vi "KE6517_Test.vi"(8 "error in (no error)":errorcluster, 11 "KE6517 in":refnum<class "KE6517.lvclass">) -> (0 "error out":errorcluster, 3 "KE6517 out":refnum<class "KE6517.lvclass">)   [LabVIEW 2013, in "KE6517.lvclass"]
uses:
  KE6517.lvclass
  <vilib>/Platform/TimedLoop/XDataNode/timing_clust.ctl
  <vilib>/Platform/TimedLoop/XDataNode/nitl_modes.ctl
  <vilib>/Platform/TimedLoop/XDataNode/wakeup.ctl
  <vilib>/platform/TimedLoop/XDataNode/XDataNode.xnode
  <vilib>/Platform/TimedLoop/XDataNode/XDNodeRunTimeDep.lvlib
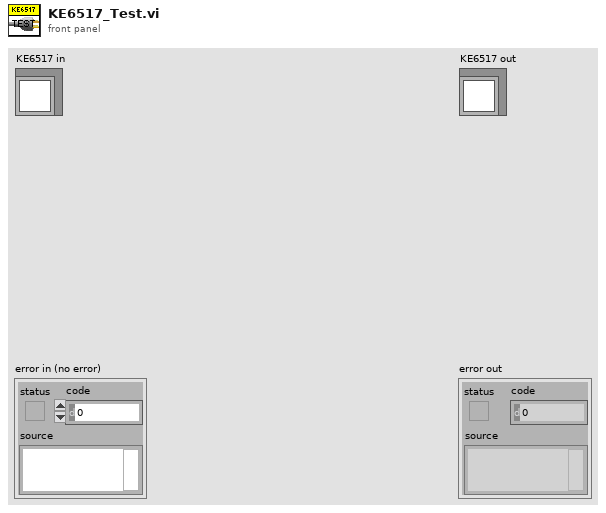
[diagram p1: front panel]
types:
  T1 = typedef "XDNodeRunTimeDep.lvlib/timing_clust.ctl" = cluster{"Expected End [f-1]":u64, "Actual End [f-1]":u64, "Finished Late? [f-1]":bool, "Expected End [i-1]":u64, "Actual End [i-1]":u64, "Finished Late? [i-1]":bool, "Expected Start [i]":u64, "Actual Start [i]":u64, "Expected Start [f]":u64, "Actual Start [f]":u64, "Source Name":string, "Structure Name":string, "Period":i64, "Deadline":i64, "Offset":i64, "Start":i64, "Priority":i32, "Timeout":i32, "Mode":T2, "Wakeup Reason":T3, "Error":errorcluster, "Source Type":string, "Secondary Source Type":string, "Global End Time":u64, "Global Start Time":u64, "Frame Duration":u64, "Iteration Duration":u64, "Assigned CPU":i32, "I/O Scan Engine Mode":u32}
  T2 = typedef "XDNodeRunTimeDep.lvlib/nitl_modes.ctl" = enum32{"No Change", "Process missed periods, maintain original phase", "Discard missed periods, maintain original phase", "Process missed periods, ignore original phase", "Discard missed periods, ignore original phase"}
  T3 = typedef "XDNodeRunTimeDep.lvlib/wakeup.ctl" = enum32{"Normal", "Aborted", "Asynchronous wakeup", "Timing source error", "Timed loop error", "Timeout"}
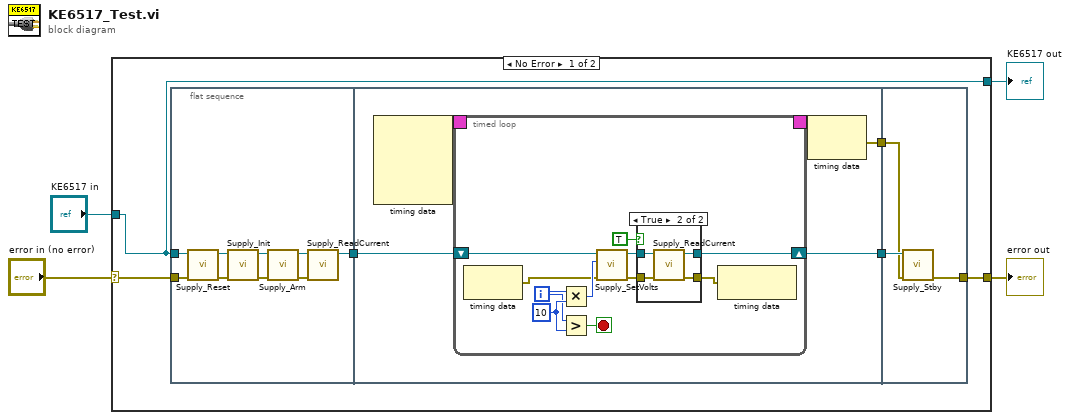
[diagram p0: block diagram]
diagram:
  n1 = case shown="No Error" "error in (no error)" {
    selector: "error in (no error)" -> [w5 w54]
    tunnel: [w7 w54] -> w3
    tunnel: [w6 w53] -> w1
    tunnel: "KE6517 in" -> [w6 w53]
    frame No Error {
      n2 = flat-sequence {
        tunnel: w5 -> [w14]
        tunnel: w6 -> [w13]
        tunnel: [w11] -> w10
        tunnel: w10 -> [w24]
        tunnel: [w23] -> w9
        tunnel: [w20] -> w8
        tunnel: [w50] -> w7
        tunnel: w9 -> [w51]
        tunnel: w8 -> [w52]
        frame #0 {
          n3 = call-dynamic "Supply_Reset.vi"("error in (no error)"=w14, "SupplyControl in"=w13) -> ("error out"=w18:errorcluster, "SupplyControl out"=w12:refnum<class "KE6517.lvclass">)  [unwired: 8 in]
          n4 = call-dynamic "Supply_Init.vi"("error in (no error)"=w18, "SupplyControl in"=w12) -> ("error out"=w17:errorcluster, "SupplyControl out"=w19:refnum<class "KE6517.lvclass">)  [unwired: 8 in]
          n5 = call-dynamic "Supply_Arm.vi"("error in (no error)"=w17, "SupplyControl in"=w19) -> ("error out"=w15:errorcluster, "SupplyControl out"=w16:refnum<class "KE6517.lvclass">)  [unwired: 8 in]
          n6 = call-dynamic "Supply_ReadCurrent.vi"("error in (no error)"=w15, "SupplyControl in"=w16) -> ("SupplyControl out"=w11:refnum<class "KE6517.lvclass">)  [unwired: 7 in, 2 out]
        }
        frame #1 {
          n7 = node-c288() -> (w22:T1)  [unwired: 4 in]
          n8 = timed-loop {
            timing: w22 -> [_]
            timing-out: [_] -> w21
            shift-right: [w32] -> w20
            shift-left: w24 -> [w29]
            i -> [w34]
            stop <- w33 stop-if-true
            w35 = 10
            n9 = node-c288() -> (w27:errorcluster)  [unwired: 1 in]
            n10 = Multiply(x=w34, y=w35) -> (x*y=w28:i32)
            n11 = Greater?(x=w34, y=w35) -> (0:w33:bool)
            n12 = call-dynamic "Supply_SetVolts.vi"("error in (no error)"=w27, "Volts IN [V]"=w28, "KE6517 in"=w29) -> ("error out"=w25:errorcluster, "KE6517 out"=w26:refnum<class "KE6517.lvclass">)  [unwired: 6 in, 1 out]
            n13 = case shown="True" TRUE {
              tunnel: w25 -> [w37 w41]
              tunnel: w26 -> [w36 w40]
              tunnel: [w36 w39] -> w32
              tunnel: [w37 w38] -> w31
              frame False {
              }
              frame True {
                n14 = call-dynamic "Supply_ReadCurrent.vi"("error in (no error)"=w41, "SupplyControl in"=w40) -> ("error out"=w38:errorcluster, "SupplyControl out"=w39:refnum<class "KE6517.lvclass">)  [unwired: 7 in, 1 out]
              }
            }
            n15 = node-c288(w31) -> ()  [unwired: 1 out]
          }
          n16 = node-c288(w21) -> (w23:errorcluster)
        }
        frame #2 {
          n17 = call-dynamic "Supply_Stby.vi"("error in (no error)"=w51, "SupplyControl in"=w52) -> ("error out"=w50:errorcluster)  [unwired: 8 in, 1 out]
        }
      }
    }
    frame Error {
    }
  }
  "error out" <- w3
  "KE6517 out" <- w1
